vi "Parser_0xEA_(SubVI).vi"(11 "String in":string) -> (2 "float number":sgl, 3 "NParam":i32)   [LabVIEW 2017, in "LV_Unicorn.lvlib"]
uses:
  LV_Unicorn.lvlib
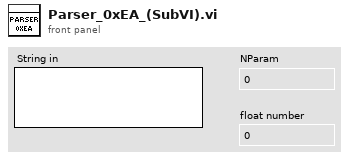
[diagram p1: front panel]
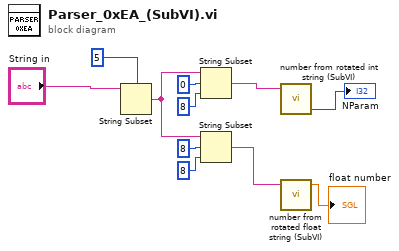
[diagram p0: block diagram]
diagram:
  n1 = String Subset(string="String in", offset (0)=5) -> (substring=w3:string)  [unwired: 1 in]
  n2 = String Subset(string=w3, offset (0)=0, length (rest)=8 ("length (rest)")) -> (substring=w9:string)
  n3 = String Subset(string=w3, offset (0)=8, length (rest)=8 ("length (rest)")) -> (substring=w2:string)
  n4 = call "number from rotated int string (SubVI).vi"("String"=w9) -> ("int number"=→"NParam":i32)  [unwired: 2 in, 2 out]
  n5 = call "number from rotated float string (SubVI).vi"("String"=w2) -> ("rotated float number"=→"float number":sgl)  [unwired: 2 in, 2 out]
